vi "DownsampleStage2_5761_10MHzPID.vi"(6 "Count to skip":u32=22, 8 "valid in":bool, 9 "reset":bool, 11 "Data in":fxp<+/-,32,14>[](array[numeric])=[0.0, 0.0, 0.0, 0.0, 0.0, 0.0, 0.0, 0.0, 0.0, 0.0]) -> (0 "valid out":bool, 3 "data out":fxp<+/-,32,14>[](array[numeric]))   [LabVIEW 2018]
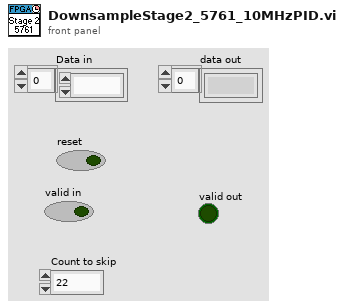
[diagram p1: front panel]
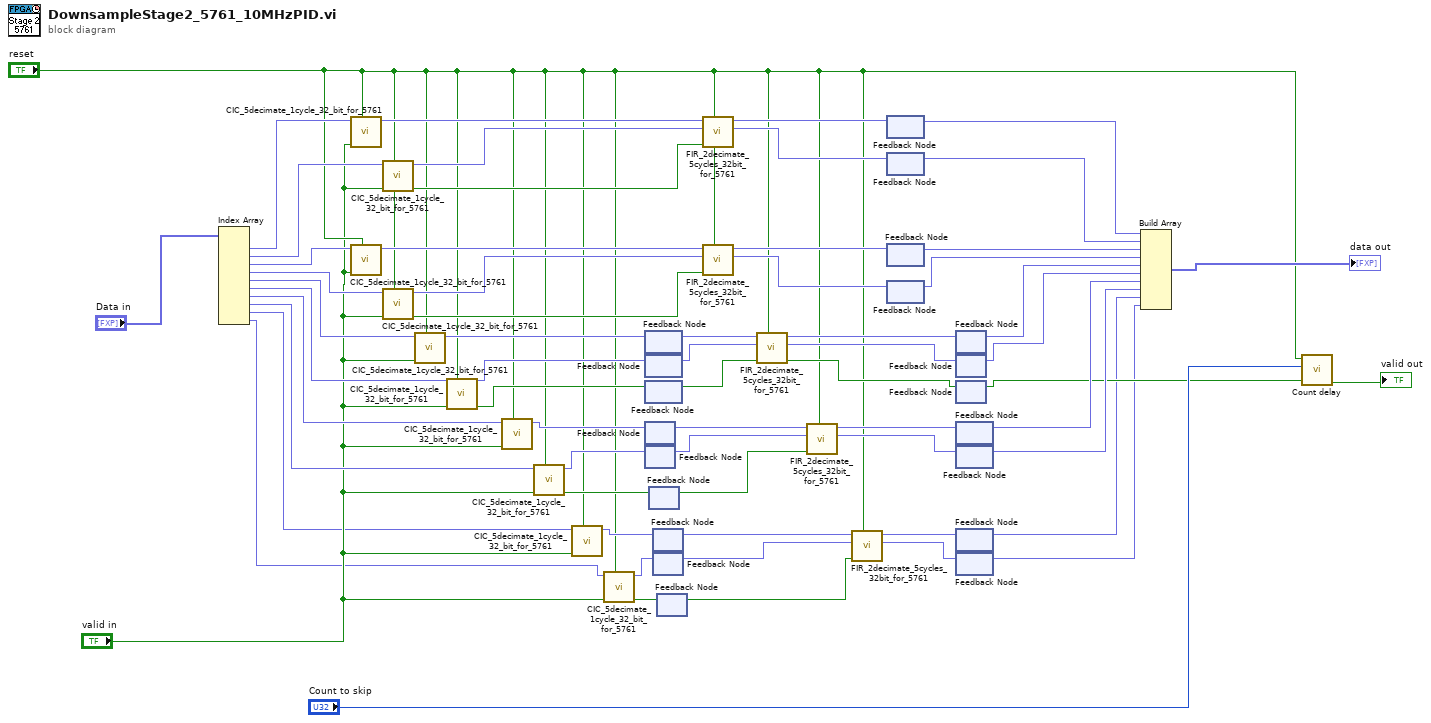
[diagram p0: block diagram]
diagram:
  n1 = Index Array(array="Data in") -> (element #1=w22:fxp<+/-,32,14>, element #2=w21:fxp<+/-,32,14>, element #3=w61:fxp<+/-,32,14>, element #4=w59:fxp<+/-,32,14>, element #5=w58:fxp<+/-,32,14>, element #6=w57:fxp<+/-,32,14>, element #7=w38:fxp<+/-,32,14>, element #8=w37:fxp<+/-,32,14>, element #9=w2:fxp<+/-,32,14>, element #10=w1:fxp<+/-,32,14>)  [unwired: 10 in]
  n2 = call "CIC_5decimate_1cycle_32_bit_for_5761.vi"("reset"="reset", "valid in"="valid in", "Data in"=w22) -> ("Data out"=w23:fxp<+/-,32,14>)  [unwired: 7 in, 1 out]
  n3 = call "CIC_5decimate_1cycle_32_bit_for_5761.vi"("reset"="reset", "valid in"="valid in", "Data in"=w61) -> ("Data out"=w50:fxp<+/-,32,14>)  [unwired: 7 in, 1 out]
  n4 = call "CIC_5decimate_1cycle_32_bit_for_5761.vi"("reset"="reset", "valid in"="valid in", "Data in"=w21) -> ("valid out"=w20:bool, "Data out"=w24:fxp<+/-,32,14>)  [unwired: 7 in]
  n5 = call "CIC_5decimate_1cycle_32_bit_for_5761.vi"("reset"="reset", "valid in"="valid in", "Data in"=w59) -> ("valid out"=w48:bool, "Data out"=w49:fxp<+/-,32,14>)  [unwired: 7 in]
  n6 = call "CIC_5decimate_1cycle_32_bit_for_5761.vi"("reset"="reset", "valid in"="valid in", "Data in"=w58) -> ("Data out"=w56:fxp<+/-,32,14>)  [unwired: 7 in, 1 out]
  n7 = call "CIC_5decimate_1cycle_32_bit_for_5761.vi"("reset"="reset", "valid in"="valid in", "Data in"=w57) -> ("valid out"=w54:bool, "Data out"=w55:fxp<+/-,32,14>)  [unwired: 7 in]
  n8 = call "CIC_5decimate_1cycle_32_bit_for_5761.vi"("reset"="reset", "valid in"="valid in", "Data in"=w38) -> ("Data out"=w32:fxp<+/-,32,14>)  [unwired: 7 in, 1 out]
  n9 = call "CIC_5decimate_1cycle_32_bit_for_5761.vi"("reset"="reset", "valid in"="valid in", "Data in"=w37) -> ("valid out"=w28:bool, "Data out"=w31:fxp<+/-,32,14>)  [unwired: 7 in]
  n10 = call "CIC_5decimate_1cycle_32_bit_for_5761.vi"("reset"="reset", "valid in"="valid in", "Data in"=w2) -> ("Data out"=w12:fxp<+/-,32,14>)  [unwired: 7 in, 1 out]
  n11 = call "CIC_5decimate_1cycle_32_bit_for_5761.vi"("reset"="reset", "valid in"="valid in", "Data in"=w1) -> ("valid out"=w14:bool, "Data out"=w13:fxp<+/-,32,14>)  [unwired: 7 in]
  n12 = feedback #1() -> (w53:fxp<+/-,32,14>)  [unwired: 1 in]
  n13 = feedback-in #1(w56) -> ()
  n14 = feedback #2() -> (w52:fxp<+/-,32,14>)  [unwired: 1 in]
  n15 = feedback-in #2(w55) -> ()
  n16 = feedback #3() -> (w51:bool)  [unwired: 1 in]
  n17 = feedback-in #3(w54) -> ()
  n18 = feedback #4() -> (w33:fxp<+/-,32,14>)  [unwired: 1 in]
  n19 = feedback-in #4(w32) -> ()
  n20 = feedback #5() -> (w34:fxp<+/-,32,14>)  [unwired: 1 in]
  n21 = feedback-in #5(w31) -> ()
  n22 = feedback #6() -> (w27:bool)  [unwired: 1 in]
  n23 = feedback-in #6(w28) -> ()
  n24 = feedback #7() -> (w9:fxp<+/-,32,14>)  [unwired: 1 in]
  n25 = feedback-in #7(w12) -> ()
  n26 = feedback #8() -> (w8:fxp<+/-,32,14>)  [unwired: 1 in]
  n27 = feedback-in #8(w13) -> ()
  n28 = feedback #9() -> (w7:bool)  [unwired: 1 in]
  n29 = feedback-in #9(w14) -> ()
  n30 = call "FIR_2decimate_5cycles_32bit_for_5761.vi"("reset"="reset", "valid in"=w20, "Q in"=w24, "I in"=w23) -> ("Q out"=w26:fxp<+/-,32,14>, "I out"=w25:fxp<+/-,32,14>)  [unwired: 4 in, 2 out]
  n31 = call "FIR_2decimate_5cycles_32bit_for_5761.vi"("reset"="reset", "valid in"=w48, "Q in"=w49, "I in"=w50) -> ("Q out"=w46:fxp<+/-,32,14>, "I out"=w47:fxp<+/-,32,14>)  [unwired: 4 in, 2 out]
  n32 = call "FIR_2decimate_5cycles_32bit_for_5761.vi"("reset"="reset", "valid in"=w51, "Q in"=w52, "I in"=w53) -> ("valid out"=w41:bool, "Q out"=w42:fxp<+/-,32,14>, "I out"=w43:fxp<+/-,32,14>)  [unwired: 4 in, 1 out]
  n33 = call "FIR_2decimate_5cycles_32bit_for_5761.vi"("reset"="reset", "valid in"=w27, "Q in"=w34, "I in"=w33) -> ("Q out"=w36:fxp<+/-,32,14>, "I out"=w35:fxp<+/-,32,14>)  [unwired: 4 in, 2 out]
  n34 = call "FIR_2decimate_5cycles_32bit_for_5761.vi"("reset"="reset", "valid in"=w7, "Q in"=w8, "I in"=w9) -> ("Q out"=w6:fxp<+/-,32,14>, "I out"=w10:fxp<+/-,32,14>)  [unwired: 4 in, 2 out]
  n35 = feedback #10() -> (w19:fxp<+/-,32,14>)  [unwired: 1 in]
  n36 = feedback-in #10(w25) -> ()
  n37 = feedback #11() -> (w18:fxp<+/-,32,14>)  [unwired: 1 in]
  n38 = feedback-in #11(w26) -> ()
  n39 = feedback #12() -> (w45:fxp<+/-,32,14>)  [unwired: 1 in]
  n40 = feedback-in #12(w47) -> ()
  n41 = feedback #13() -> (w44:fxp<+/-,32,14>)  [unwired: 1 in]
  n42 = feedback-in #13(w46) -> ()
  n43 = feedback #14() -> (w39:fxp<+/-,32,14>)  [unwired: 1 in]
  n44 = feedback-in #14(w43) -> ()
  n45 = feedback #15() -> (w40:fxp<+/-,32,14>)  [unwired: 1 in]
  n46 = feedback-in #15(w42) -> ()
  n47 = feedback #16() -> (w16:bool)  [unwired: 1 in]
  n48 = feedback-in #16(w41) -> ()
  n49 = feedback #17() -> (w30:fxp<+/-,32,14>)  [unwired: 1 in]
  n50 = feedback-in #17(w35) -> ()
  n51 = feedback #18() -> (w29:fxp<+/-,32,14>)  [unwired: 1 in]
  n52 = feedback-in #18(w36) -> ()
  n53 = feedback #19() -> (w5:fxp<+/-,32,14>)  [unwired: 1 in]
  n54 = feedback-in #19(w10) -> ()
  n55 = feedback #20() -> (w4:fxp<+/-,32,14>)  [unwired: 1 in]
  n56 = feedback-in #20(w6) -> ()
  n57 = Build Array(w19, w18, w45, w44, w39, w40, w30, w29, w5, w4) -> (→"data out":fxp<+/-,32,14>[])
  n58 = call "Count delay.vi"("input valid"=w16, "Count to skip"="Count to skip", "Reset"="reset") -> ("output valid"=→"valid out":bool)  [unwired: 7 in, 1 out]
